vi "Get DDG Step Coefficients.vi"(9 "p2":dbl, 10 "p1":dbl, 11 "mode":u32) -> (1 "p2 out":dbl, 2 "p1 out":dbl, 3 "function return":u32)   [LabVIEW 2018, in "Copy of Andor SDK.lvlib"]
doc: "EXPNETTYPE unsigned int WINAPI GetDDGStepCoefficients(at_u32 mode, double * p1, double * p2);"
uses:
  Copy of Andor SDK.lvlib
  <userlib>/Andor SDK/ATMCD32D.dll
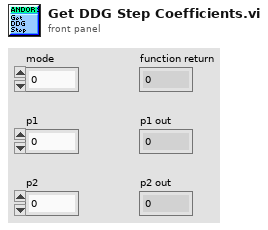
[diagram p1: front panel]
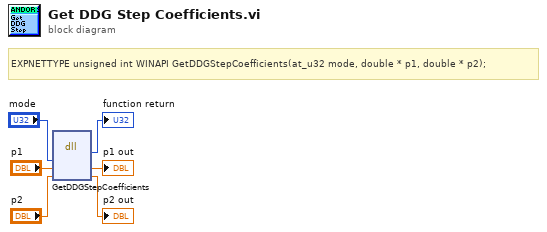
[diagram p0: block diagram]
diagram:
  # "EXPNETTYPE unsigned int WINAPI GetDDGStepCoefficients(at_u32 mode, double * p1, double * p2);"
  n1 = dll-call lib="C:/Program Files (x86)/National Instruments/LabVIEW 2018/user.lib/Andor SDK/ATMCD32D.*" fn="GetDDGStepCoefficients"("mode"="mode", "p1"="p1", "p2"="p2") -> (→"function return":u32, "p1"=→"p1 out":dbl, "p2"=→"p2 out":dbl)  [unwired: 4 in, 2 out]
